vi "Vi_por_infeite_deletar_depois.vi"(8 "Numeric 5":dbl, 9 "Numeric 2":dbl, 10 "Numeric":dbl) -> (1 "Numeric 4":dbl, 2 "Numeric 3":dbl, 3 "Boolean":bool)   [LabVIEW 2020]
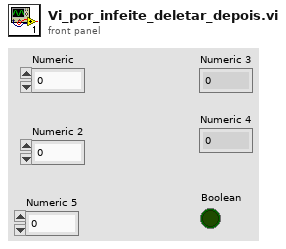
[diagram p1: front panel]
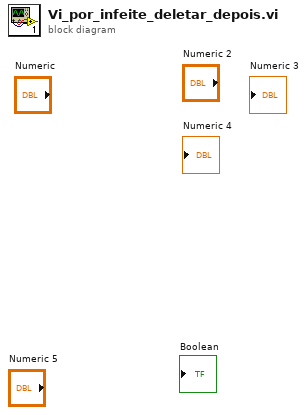
[diagram p0: block diagram]
diagram:
